vi "Generate Single line AO sequence.vi"(11 "Variables":T1 {"Dwell time" format="%#_6f"; "Sample Clock Rate" format="%#_6f"}) -> (2 "Single line AO sequence":dbl[](array[numeric]))   [LabVIEW 2020]
uses:
  Typedefs/Pockels mod gen variables cluster.ctl
  Typedefs/Imaging Protocols enum.ctl
  Typedefs/Rounding type.ctl
  Globals/gl_Pockels control globals.vi
panel:
  out "Full sequence (points)":i32
  out "Length of sequence (ms)":dbl format="%#_6f"
  out "Single line pockels modulation waveform":dbl[](graph)
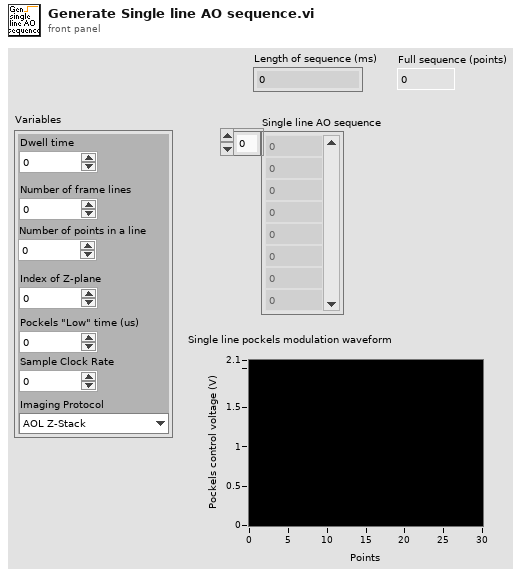
[diagram p1: front panel]
types:
  T1 = typedef "Pockels mod gen variables cluster.ctl" = cluster{"Dwell time":dbl, "Number of frame lines":i32, "Number of points in a line":i32, "Index of Z-plane":i32, "Pockels \"Low\" time (us)":dbl, "Sample Clock Rate":dbl, "Imaging Protocol":T2}
  T2 = typedef "Imaging Protocols enum.ctl" = enum16{"AOL Z-Stack", "Motor Z Stack", "Functional Acquisition", "Single Plane Acquisition", "Volume Acquisition", "Live Imaging", "Live Plane Imaging", "Live Volume Imaging"}
  T3 = typedef "Rounding type.ctl" = enum16{"No rounding", "Toward +Inf", "Toward -Inf"}
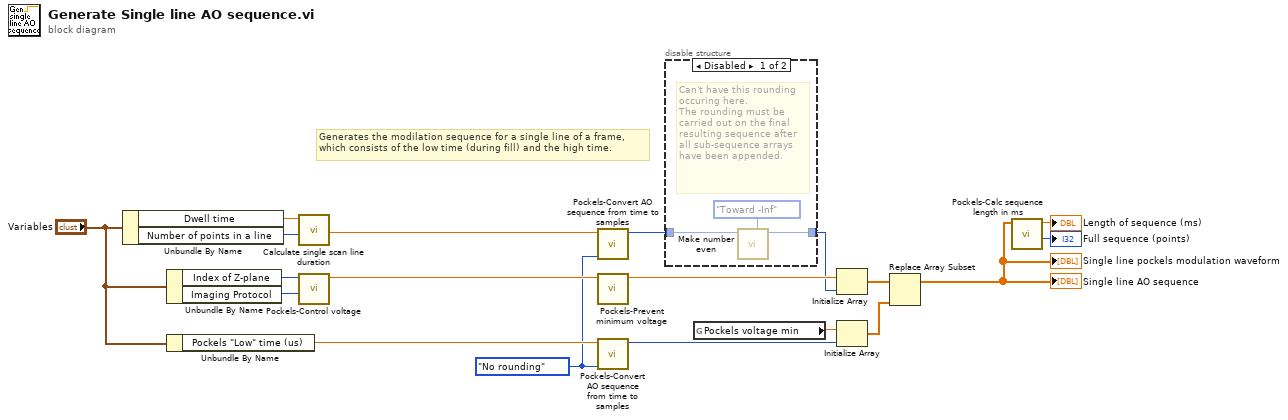
[diagram p0: block diagram]
diagram:
  w1 = Rounding_type."No rounding" ("Direction (+Inf)")
  # "Generates the modilation sequence for a single line of a frame,\nwhich consists of the low time (during fill) and the high time."
  n1 = Unbundle By Name("Variables") -> ("Dwell time"=w10:dbl, "Number of points in a line"=w9:i32)
  n2 = Unbundle By Name("Variables") -> ("Index of Z-plane"=w8:i32, "Imaging Protocol"=w7:T2)
  n3 = Unbundle By Name("Variables") -> ("Pockels \"Low\" time (us)"=w5:dbl)
  n4 = call "Calculate single scan line duration.vi"("Points in a scan line (~frame size)"=w9, "Dwell time (us)"=w10) -> ("Line scan time (us)"=w16:dbl)  [unwired: 9 in]
  n5 = call "Pockels-Control voltage.vi"("Imaging Protocol"=w7, "Index of Z-plane"=w8) -> ("Pockels control voltage (V)"=w17:dbl)  [unwired: 8 in, 1 out]
  n6 = call "Pockels-Convert AO sequence from time to samples.vi"("Direction (+Inf)"=w1, "Duration of AO sequence (us)"=w16) -> ("Number of samples in AO sequence"=w14:i32)  [unwired: 9 in]
  n7 = call "Pockels-Prevent minimum voltage.vi"("Pockels Value"=w17) -> ("Pockels Value (minimum prevented)"=w18:dbl)  [unwired: 8 in, 2 out]
  n8 = call "Pockels-Convert AO sequence from time to samples.vi"("Direction (+Inf)"=w1, "Duration of AO sequence (us)"=w5) -> ("Number of samples in AO sequence"=w12:i32)  [unwired: 9 in]
  n9 = disable-structure shown="Disabled" {
    disable-tunnel: w14 -> [w22 w23]
    disable-tunnel: [w20 w23] -> w13
    frame Disabled {
      # "Can't have this rounding occuring here.\nThe rounding must be carried out on the final resulting sequence after all sub-sequence arrays have been appended."
      n10 = call <userlib>:"Make number even.vi"("Direction (+Inf)"=enum16{"Toward +Inf", "Toward -Inf"}."Toward -Inf", "Number in"=w22) -> ("Even number"=w20:i32)  [unwired: 9 in]
    }
    frame Enabled {
    }
  }
  n11 = global read "gl_Pockels control globals.vi" "Pockels voltage min"() -> (w15:dbl)
  n12 = Initialize Array(w18, w13) -> (w11:dbl[])
  n13 = Initialize Array(w15, w12) -> (w19:dbl[])
  n14 = Replace Array Subset "Replace Array Subset"(array=w11, new element=w19) -> (w3:dbl[])  [unwired: 1 in]
  "Single line AO sequence" <- w3
  "Single line pockels modulation waveform" <- w3
  n15 = call "Pockels-Calc sequence length in ms.vi"("Pockels modulation sequence in"=w3) -> ("Sequence length (points)"=→"Full sequence (points)":i32, "Sequence length (ms)"=→"Length of sequence (ms)":dbl)  [unwired: 8 in, 1 out]
